vi "shag_start — 7.vi"() -> ()   [LabVIEW 2016]
uses:
  <vilib>/Instr/_visa.llb/VISA Configure Serial Port (Instr).vi
panel:
  out "file 2":string
  out "положение в мин 2":i32
  out "file":i32
  out "положение в мин 1":i32
  in  "all":T1(tab)
  out "положение шд 2":i32(knob) scale=-10.0..190.0
  out "текущее положение 2":string
  out "положение в минутах 2":string
  in  "Минуты 2":i32 min=-600 max=11400
  in  "Stop двигатель 2":bool
  in  "Вращение по градусам +  2":bool
  in  "Вращение по градусам -  2":bool
  in  "Вернуться в нулевое положение 2":bool
  in  "Задать текущее положение нулевым 2":bool
  in  "Установка минут 2":bool
  in  "Блокировать трубку №2":bool
  out "положение шд":i32(knob) scale=-10.0..190.0
  out "текущее положение":string
  out "положение в минутах 1":string
  in  "Минуты":i32 min=-600 max=11400
  in  "Stop двигатель":bool
  in  "Вращение по градусам +":bool
  in  "Вращение по градусам -":bool
  in  "Вернуться в нулевое положение":bool
  in  "Задать текущее положение нулевым":bool
  in  "Установка минут":bool
  in  "Блокировать зеркало №1":bool
  in  "stop":bool
  in  "Выберете COM порт":refnum<visa-resource-name>="COM1"
  in  "Скорость обмена данными":u32(ring)=19200 items=["9600"=9600, "19200"=19200, "38400"=38400, "57600"=57600]
  in  "Число бит на символ":u16=8 min=5 max=8 step=1
  in  "Контроль чётности":enum16{"None", "Odd", "Even", "Mark", "Space"}(ring)
  in  "Стоповый бит":u16(ring)=10 items=["1.0"=10, "1.5"=15, "2.0"=20]
  in  "Контроль переполнения":u16(ring) items=["None"=0, "XON/XOFF"=1, "RTS/CTS"=2, "DTR/DSR"=4]
  # "1 - адресс 1 двигателя\n2 - адресс 2 двигателя\n$0MV\\01+   - запуск всех двигателей в положительном направлении \n$0MS\\00   - остановка всех двигателей\n$0MJ\\04+\\00\\00\\01   - 1 шаг всех двигателей\n$0SS\\01\\10   - скорость 10 для всех двигателей"
  # "Ренгеновская трубка №2"
  # "Положение:"
  # "Зеркало №1"
  # "Положение:"
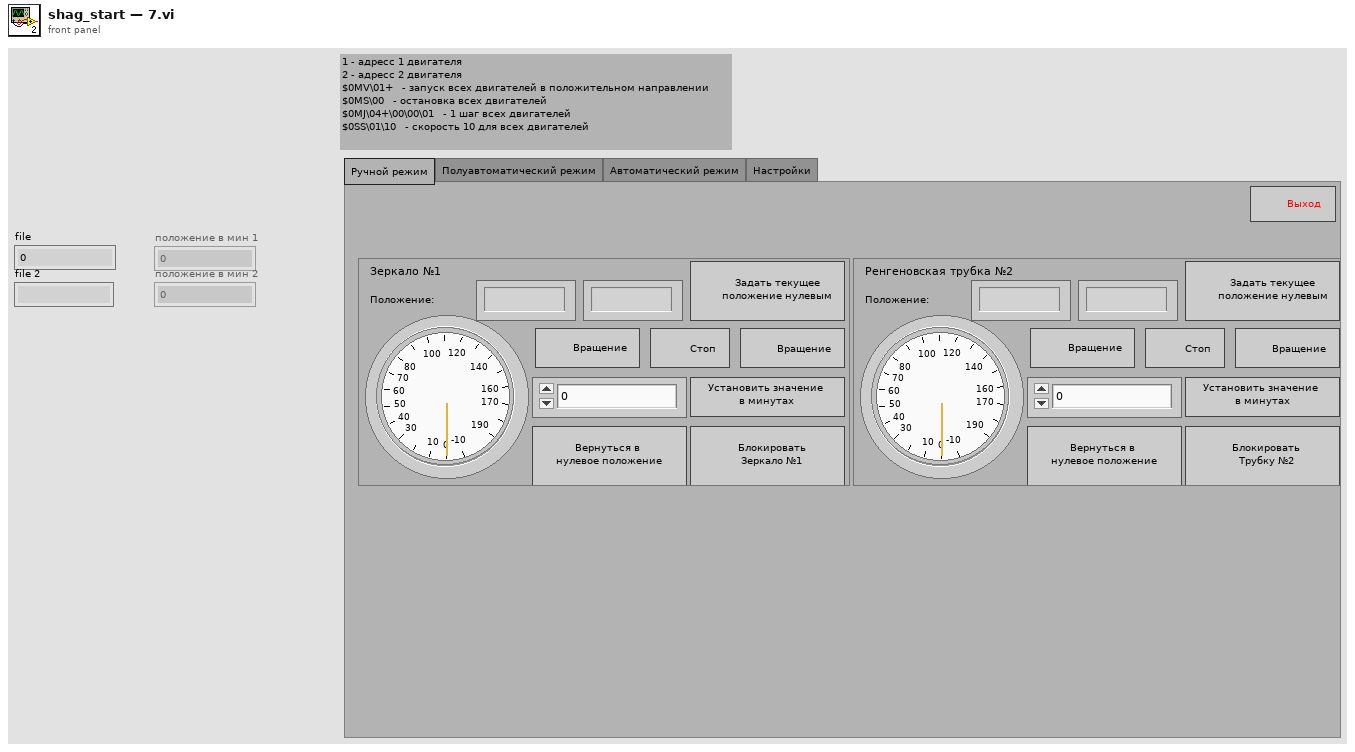
[diagram p1: front panel]
types:
  T1 = enum32{"Ручной режим", "Полуавтоматический режим", "Автоматический режим", "Настройки"}
  T2 = enum16{"open", "replace", "create", "open or create", "replace or create", "replace or create with confirmation"}
  T3 = enum8{"Enabled", "Disabled", "Disabled and Grayed Out"}
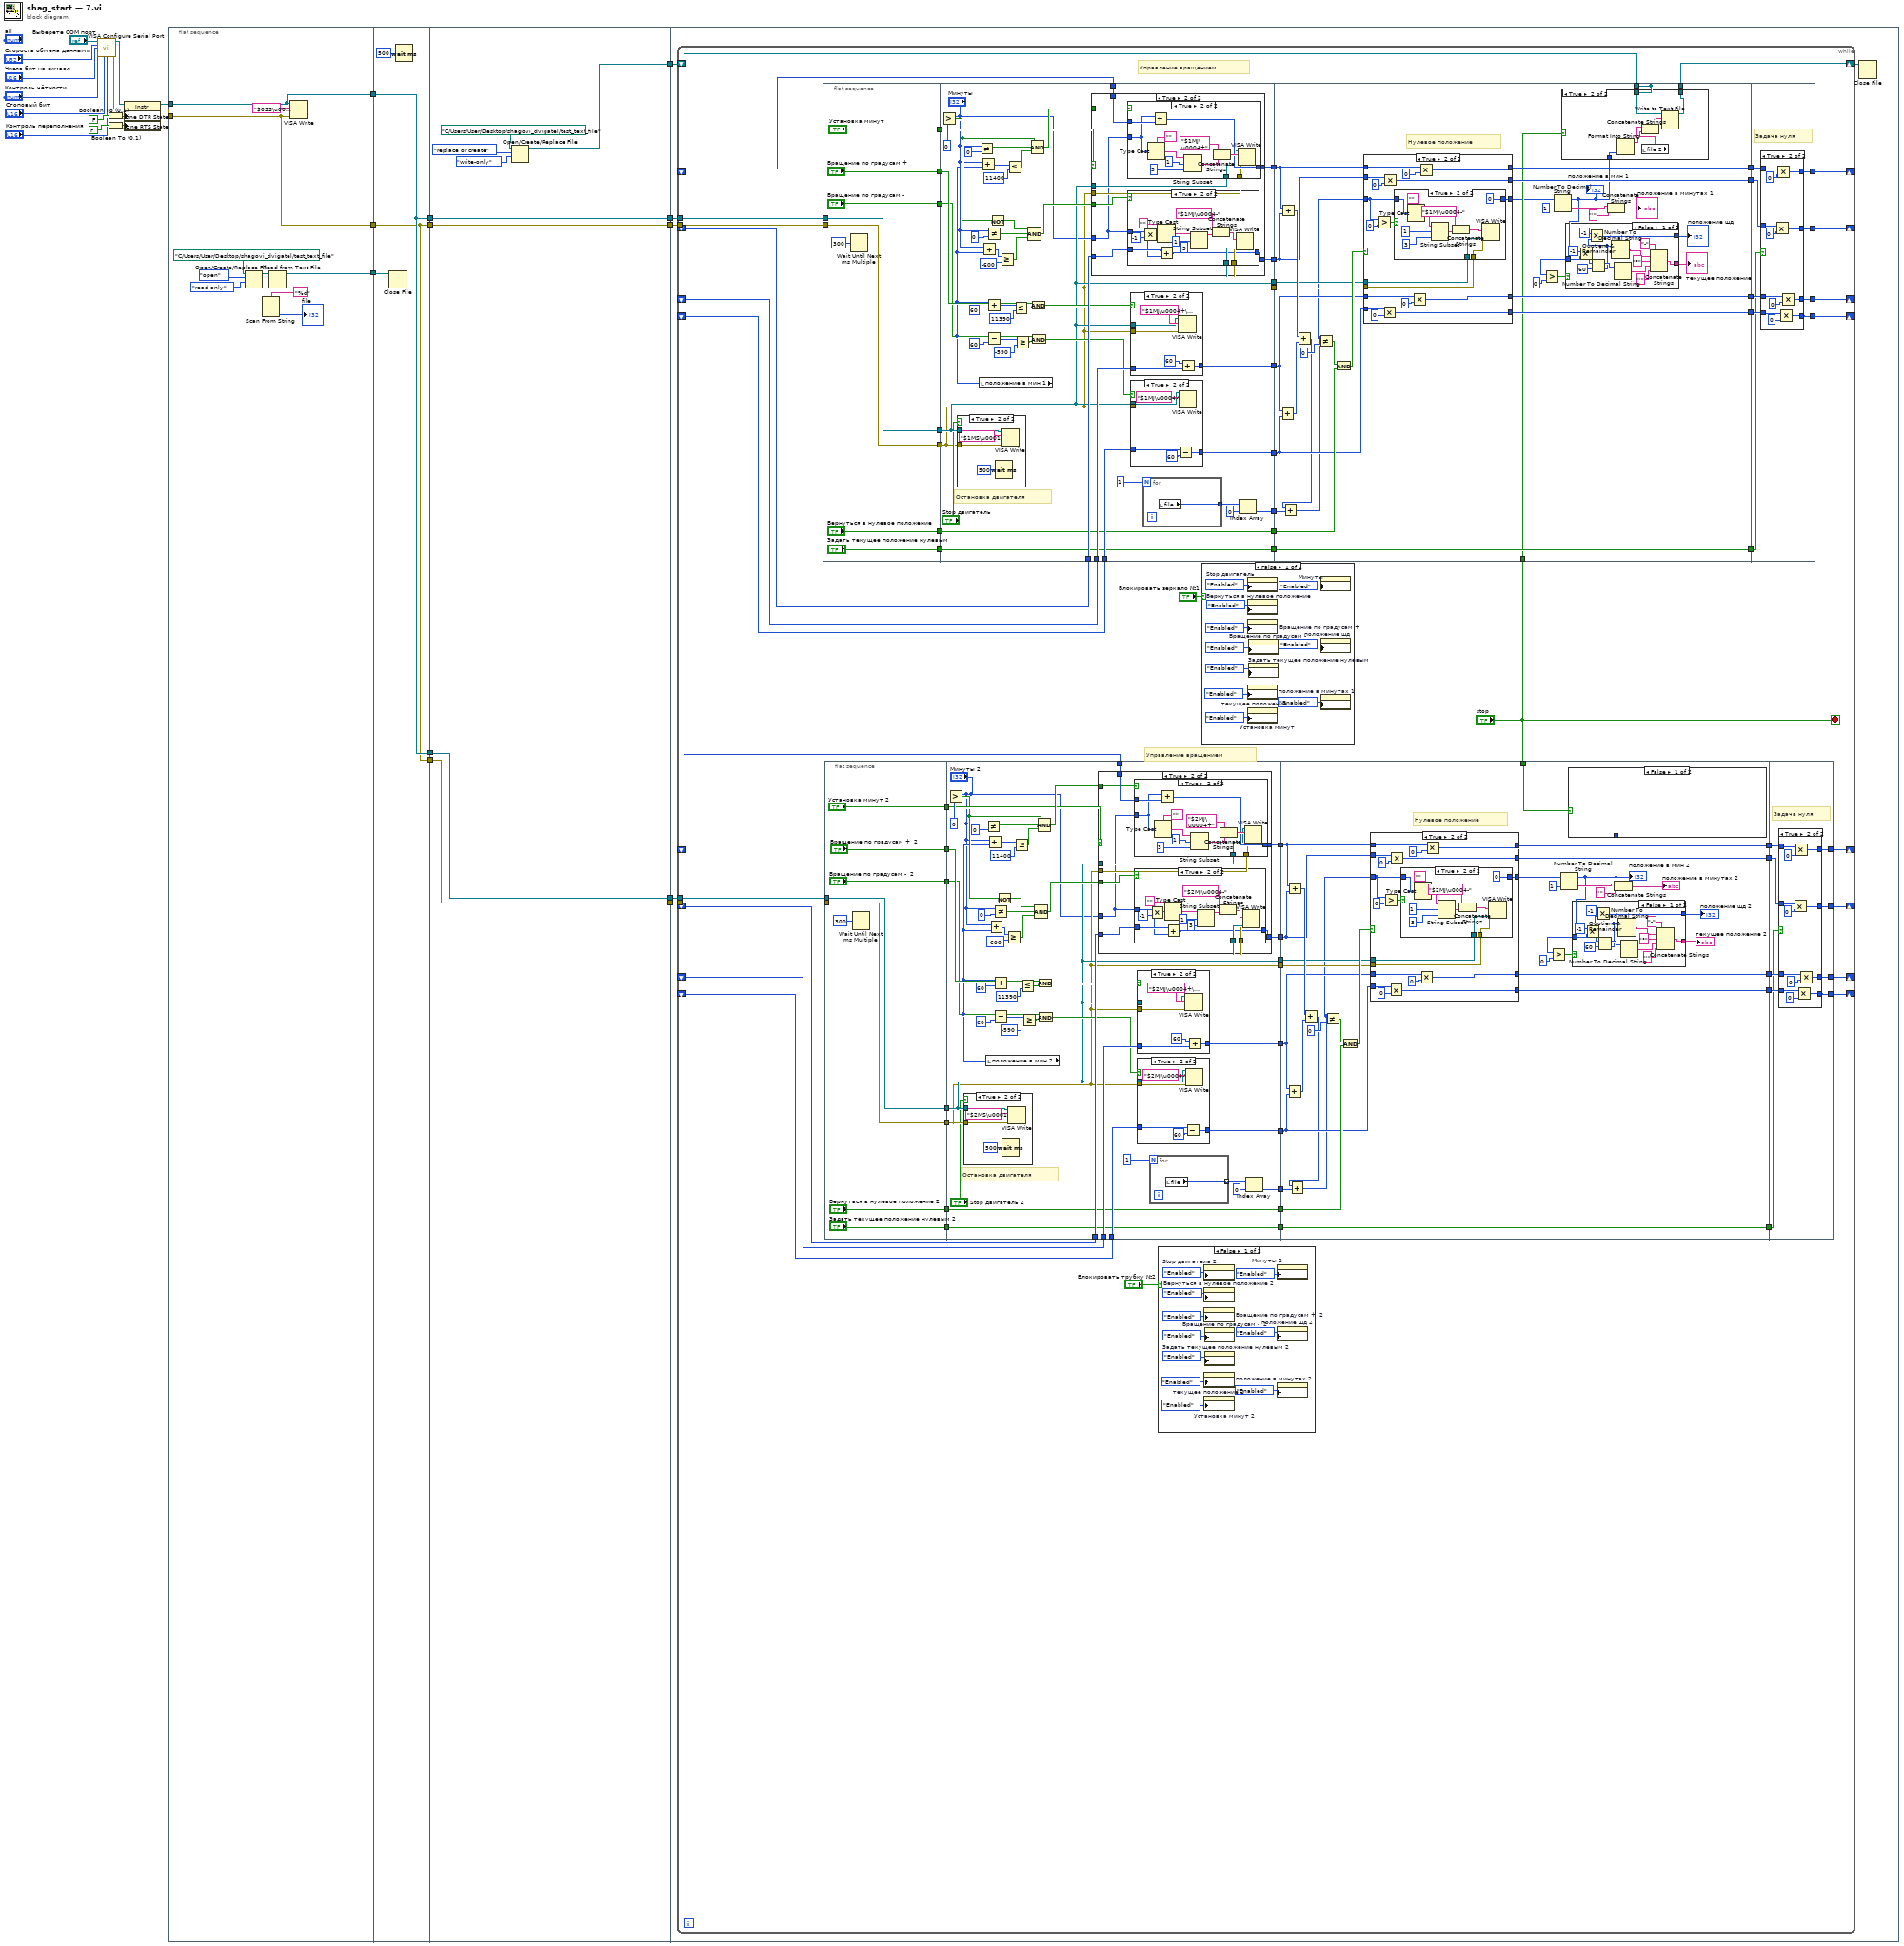
[diagram p0: block diagram]
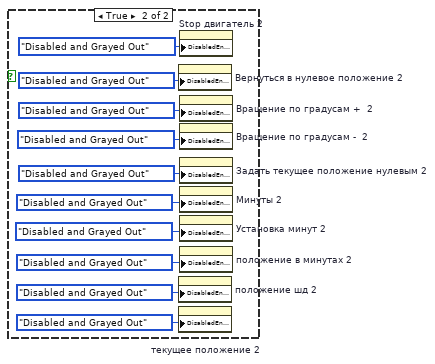
[diagram p2: hidden frame]
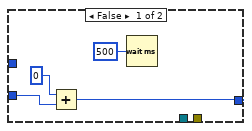
[diagram p4: hidden frame]
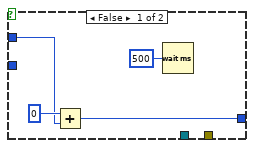
[diagram p5: hidden frame]
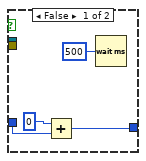
[diagram p7: hidden frame]
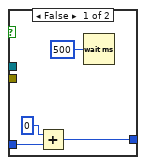
[diagram p8: hidden frame]
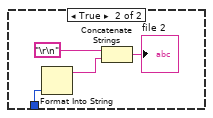
[diagram p9: hidden frame]
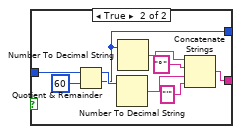
[diagram p10: hidden frame]
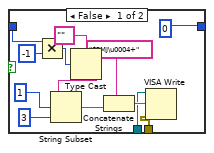
[diagram p12: hidden frame]
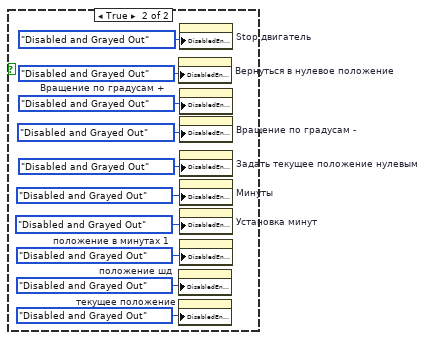
[diagram p14: hidden frame]
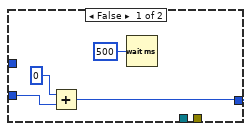
[diagram p16: hidden frame]
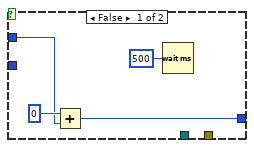
[diagram p17: hidden frame]
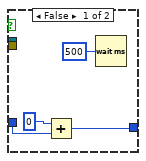
[diagram p19: hidden frame]
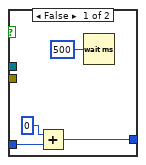
[diagram p20: hidden frame]
diagram:
  n1 = call-poly "VISA Configure Serial Port"("VISA resource name"="Выберете COM порт", "baud rate (9600)"="Скорость обмена данными", "data bits (8)"="Число бит на символ", "parity (0:none)"="Контроль чётности", "stop bits (10: 1 bit)"="Стоповый бит", "flow control (0:none)"="Контроль переполнения") -> ("VISA resource name out"=w24:refnum<visa-resource-name>, "error out"=w23:errorcluster)  [unwired: 8 in]
  n2 = Boolean To (0,1)(Boolean=FALSE ("DTR Write")) -> (0, 1=w25:i16)
  n3 = Boolean To (0,1)(Boolean=FALSE ("DTR Write")) -> (0, 1=w26:i16)
  n4 = property class="Instr"(reference=w24, error in=w23, "Serial Settings:Modem Line Settings:Line DTR State"=w25, "Serial Settings:Modem Line Settings:Line RTS State"=w26) -> (reference out=w22:refnum<visa-resource-name>, error out=w21:errorcluster)
  n5 = flat-sequence {
    tunnel: w22 -> [w36]
    tunnel: w21 -> [w35]
    tunnel: [w36] -> w20
    tunnel: [w35] -> w19
    tunnel: [w29] -> w10
    tunnel: [w40] -> w9
    tunnel: w20 -> [w40]
    tunnel: w19 -> [w39]
    tunnel: [w39] -> w7
    tunnel: [w40] -> w5
    tunnel: [w39] -> w3
    tunnel: w10 -> [w38]
    tunnel: w9 -> [w49]
    tunnel: [w49] -> w8
    tunnel: w7 -> [w48]
    tunnel: [w48] -> w6
    tunnel: w5 -> [w47]
    tunnel: [w47] -> w4
    tunnel: w3 -> [w46]
    tunnel: [w46] -> w2
    tunnel: [w42] -> w1
    tunnel: w8 -> [w55]
    tunnel: w6 -> [w54]
    tunnel: w4 -> [w50]
    tunnel: w2 -> [w53]
    tunnel: w1 -> [w52]
    frame #0 {
      n6 = Open/Create/Replace File(file path (use dialog)=path "C:/Users/User/Desktop/shagovi_dvigatel/test_text_file", operation (0:open)=T2."open", access (0:read/write)=enum16{"read/write", "read-only", "write-only"}."read-only") -> (refnum out=w28:refnum<file>)  [unwired: 3 in, 2 out]
      n7 = Read from Text File(file (use dialog)=w28) -> (refnum out=w29:refnum<file>, text=w32:string)  [unwired: 3 in, 2 out]
      n8 = Scan From String(format string="%d", input string=w32) -> (output 1=→"file":i32)  [unwired: 3 in, 3 out]
      n9 = VISA Write(VISA resource name=w36, write buffer="$0SS\u0001\u0010", error in (no error)=w35) -> ()  [unwired: 3 out]
    }
    frame #1 {
      n10 = Close File(refnum=w38) -> ()  [unwired: 1 in, 2 out]
      n11 = Wait (ms)(milliseconds to wait=u32 500) -> ()  [unwired: 1 out]
    }
    frame #2 {
      n12 = Open/Create/Replace File(file path (use dialog)=path "C:/Users/User/Desktop/shagovi_dvigatel/test_text_file", operation (0:open)=T2."replace or create", access (0:read/write)=enum16{"read/write", "read-only", "write-only"}."write-only") -> (refnum out=w42:refnum<file>)  [unwired: 3 in, 2 out]
    }
    frame #3 {
      n13 = while {
        tunnel: w55 -> [w98]
        tunnel: w54 -> [w97]
        shift-right: [w93] -> _
        shift-left: _ -> [w102]
        shift-right: [w94] -> _
        shift-left: _ -> [w101]
        shift-right: [w95] -> _
        shift-left: _ -> [w100]
        shift-right: [w96] -> _
        shift-left: _ -> [w99]
        tunnel: w53 -> [w67]
        shift-right: [w89] -> w51
        shift-left: w52 -> [w90]
        tunnel: w50 -> [w66]
        shift-right: [w62] -> _
        shift-left: _ -> [w63]
        shift-right: [w60] -> _
        shift-left: _ -> [w61]
        shift-right: [w58] -> _
        shift-left: _ -> [w59]
        shift-right: [w56] -> _
        shift-left: _ -> [w57]
        stop <- "stop" stop-if-true
        # "Управление вращением"
        # "Управление вращением"
        n14 = flat-sequence {
          tunnel: w97 -> [w423]
          tunnel: w98 -> [w424]
          tunnel: [w424] -> w122
          tunnel: [w423] -> w121
          tunnel: ["Вращение по градусам +"] -> w120
          tunnel: ["Вращение по градусам -"] -> w119
          tunnel: ["Вернуться в нулевое положение"] -> w118
          tunnel: ["Задать текущее положение нулевым"] -> w117
          tunnel: ["Установка минут"] -> w116
          tunnel: w122 -> [w448]
          tunnel: w121 -> [w430]
          tunnel: [w471] -> w115
          tunnel: w102 -> [w468]
          tunnel: w101 -> [w470]
          tunnel: [w469] -> w114
          tunnel: w100 -> [w467]
          tunnel: w99 -> [w466]
          tunnel: w120 -> [w452]
          tunnel: w119 -> [w451]
          tunnel: [w465] -> w113
          tunnel: [w464] -> w112
          tunnel: [w449] -> w111
          tunnel: w118 -> [w449]
          tunnel: [w430] -> w110
          tunnel: [w448] -> w109
          tunnel: [w447] -> w108
          tunnel: w117 -> [w447]
          tunnel: w116 -> [w441]
          tunnel: [w428] -> w91
          tunnel: w115 -> [w553]
          tunnel: w114 -> [w554]
          tunnel: [w573] -> w107
          tunnel: [w571] -> w106
          tunnel: w113 -> [w555]
          tunnel: w112 -> [w556]
          tunnel: [w562] -> w105
          tunnel: [w569] -> w104
          tunnel: w111 -> [w565]
          tunnel: w110 -> [w561]
          tunnel: w109 -> [w560]
          tunnel: w108 -> [w558]
          tunnel: [w558] -> w103
          tunnel: [w547] -> _
          tunnel: "stop" -> [w550]
          tunnel: w90 -> [w547]
          tunnel: w91 -> [w545]
          tunnel: [w542] -> w89
          tunnel: [w659] -> w93
          tunnel: [w656] -> w94
          tunnel: w107 -> [w658]
          tunnel: w106 -> [w657]
          tunnel: [w655] -> w95
          tunnel: [w654] -> w96
          tunnel: w105 -> [w653]
          tunnel: w104 -> [w652]
          tunnel: w103 -> [w651]
          frame #0 {
            n15 = Wait Until Next ms Multiple(millisecond multiple=u32 300) -> ()  [unwired: 1 out]
          }
          frame #1 {
            # "Остановка двигателя"
            n16 = Greater?(x="Минуты", y=0) -> (0:w439:bool)
            n17 = case shown="True" "Stop двигатель" {
              tunnel: w448 -> [_ w519]
              tunnel: w430 -> [_ w518]
              frame False {
              }
              frame True {
                n18 = Wait (ms)(milliseconds to wait=u32 500) -> ()  [unwired: 1 out]
                n19 = VISA Write(VISA resource name=w519, write buffer="$1MS\u0001", error in (no error)=w518) -> ()  [unwired: 3 out]
              }
            }
            n20 = Not Equal?(x="Минуты", y=0) -> (x != y?=w438:bool)
            n21 = local read "положение в мин 1"() -> (w429:i32)
            n22 = Add(x="Минуты", y=w429) -> (x+y=w462:i32)
            n23 = Add(x="Минуты", y=w429) -> (x+y=w433:i32)
            n24 = Not Equal?(x="Минуты", y=0) -> (x != y?=w436:bool)
            n25 = Add(x=w429, y=60) -> (x+y=w457:i32)
            n26 = Subtract(x=w429, y=60) -> (x-y=w444:i32)
            n27 = Not(x=w439) -> (.not. x?=w440:bool)
            n28 = Greater Or Equal?(x=w433, y=-600) -> (x >= y?=w434:bool)
            n29 = Less Or Equal?(x=w462, y=11400) -> (x <= y?=w437:bool)
            n30 = Less Or Equal?(x=w457, y=11390) -> (x <= y?=w454:bool)
            n31 = Greater Or Equal?(x=w444, y=-590) -> (x >= y?=w445:bool)
            n32 = Compound Arithmetic op=AND(w440, w436, w434) -> (w458:bool)
            n33 = And(x=w452, y=w454) -> (x .and. y?=w453:bool)
            n34 = And(x=w451, y=w445) -> (x .and. y?=w450:bool)
            n35 = Compound Arithmetic op=AND(w439, w438, w437) -> (w460:bool)
            n36 = case shown="True" w441 {
              tunnel: [w474 w483] -> w471
              tunnel: w470 -> [w473 w482]
              tunnel: [w473 w481] -> w469
              tunnel: w468 -> [w474 w480]
              tunnel: w460 -> [_ w479]
              tunnel: w458 -> [_ w478]
              tunnel: w430 -> [_ w477]
              tunnel: w448 -> [_ w476]
              tunnel: "Минуты" -> [_ w475]
              frame False {
              }
              frame True {
                n37 = case shown="True" w479 {
                  tunnel: [w504 w510] -> w483
                  tunnel: w480 -> [w503 w509]
                  tunnel: w477 -> [_ w508]
                  tunnel: w476 -> [_ w507]
                  tunnel: w475 -> [_ w506]
                  frame False {
                    n38 = Add(x=0, y=w503) -> (x+y=w504:i32)
                    n39 = Wait (ms)(milliseconds to wait=u32 500) -> ()  [unwired: 1 out]
                  }
                  frame True {
                    n40 = Type Cast(type="", x=w506) -> (*(type *) &x=w513:string)
                    n41 = Add(x=w506, y=w509) -> (x+y=w510:i32)
                    n42 = String Subset(string=w513, offset (0)=1, length (rest)=3 ("length (rest)")) -> (substring=w512:string)
                    n43 = Concatenate Strings("$1MJ\u0004+" ("write buffer"), w512) -> (w516:string)
                    n44 = VISA Write(VISA resource name=w507, write buffer=w516, error in (no error)=w508) -> ()  [unwired: 3 out]
                  }
                }
                n45 = case shown="True" w478 {
                  tunnel: [w486 w492] -> w481
                  tunnel: w482 -> [w485 w491]
                  tunnel: w476 -> [_ w494]
                  tunnel: w477 -> [_ w493]
                  tunnel: w475 -> [_ w488]
                  frame False {
                    n46 = Add(x=0, y=w485) -> (x+y=w486:i32)
                    n47 = Wait (ms)(milliseconds to wait=u32 500) -> ()  [unwired: 1 out]
                  }
                  frame True {
                    n48 = Multiply(x=w488, y=-1) -> (x*y=w490:i32)
                    n49 = Type Cast(type="", x=w490) -> (*(type *) &x=w497:string)
                    n50 = Add(x=w491, y=w488) -> (x+y=w492:i32)
                    n51 = String Subset(string=w497, offset (0)=1, length (rest)=3 ("length (rest)")) -> (substring=w496:string)
                    n52 = Concatenate Strings("$1MJ\u0004-" ("write buffer"), w496) -> (w500:string)
                    n53 = VISA Write(VISA resource name=w494, write buffer=w500, error in (no error)=w493) -> ()  [unwired: 3 out]
                  }
                }
              }
            }
            n54 = case shown="True" w453 {
              tunnel: [w534 w541] -> w465
              tunnel: w467 -> [w533 w536]
              tunnel: w448 -> [_ w537]
              tunnel: w430 -> [_ w538]
              frame False {
                n55 = Add(x=0, y=w533) -> (x+y=w534:i32)
                n56 = Wait (ms)(milliseconds to wait=u32 500) -> ()  [unwired: 1 out]
              }
              frame True {
                n57 = VISA Write(VISA resource name=w537, write buffer="$1MJ\u0004+\u0000\u0000<", error in (no error)=w538) -> ()  [unwired: 3 out]
                n58 = Add(x=60, y=w536) -> (x+y=w541:i32)
              }
            }
            n59 = case shown="True" w450 {
              tunnel: [w524 w527] -> w464
              tunnel: w466 -> [w523 w526]
              tunnel: w448 -> [_ w530]
              tunnel: w430 -> [_ w529]
              frame False {
                n60 = Add(x=0, y=w523) -> (x+y=w524:i32)
                n61 = Wait (ms)(milliseconds to wait=u32 500) -> ()  [unwired: 1 out]
              }
              frame True {
                n62 = Subtract(x=w526, y=60 ("x")) -> (x-y=w527:i32)
                n63 = VISA Write(VISA resource name=w530, write buffer="$1MJ\u0004-\u0000\u0000<", error in (no error)=w529) -> ()  [unwired: 3 out]
              }
            }
            n64 = for {
              N: 1 -> [_]
              tunnel: [w472] -> w426 mode=indexing
              n65 = local read "file"() -> (w472:i32)
            }
            n66 = Index Array(array=w426, index=0) -> (element=w428:i32)
          }
          frame #2 {
            # "Нулевое положение"
            n67 = Add(x=w555, y=w556) -> (x+y=w566:i32)
            n68 = Add(x=w553, y=w554) -> (x+y=w570:i32)
            n69 = Add(x=w570, y=w566) -> (x+y=w544:i32)
            n70 = Add(x=w544, y=w545) -> (x+y=w543:i32)
            n71 = Not Equal?(x=w543, y=0 ("x")) -> (x != y?=w563:bool)
            n72 = And(x=w563, y=w565) -> (x .and. y?=w572:bool)
            n73 = case shown="True" w572 {
              tunnel: [w604 w626] -> w546
              tunnel: w553 -> [w608 w623]
              tunnel: [w608 w622] -> w573
              tunnel: [w607 w621] -> w571
              tunnel: w543 -> [w604 w615]
              tunnel: [w605 w617] -> w569
              tunnel: [w606 w614] -> w562
              tunnel: w554 -> [w607 w613]
              tunnel: w561 -> [_ w612]
              tunnel: w560 -> [_ w611]
              tunnel: w555 -> [w606 w610]
              tunnel: w556 -> [w605 w609]
              frame False {
              }
              frame True {
                n74 = Greater?(x=w615, y=0) -> (0:w616:bool)
                n75 = Multiply(x=w609, y=0) -> (x*y=w617:i32)
                n76 = Multiply(x=w613, y=0) -> (x*y=w621:i32)
                n77 = case shown="True" w616 {
                  tunnel: w615 -> [w631 w644]
                  tunnel: [0 0] -> w626
                  tunnel: w611 -> [w628 w641]
                  tunnel: w612 -> [w627 w640]
                  frame False {
                    n78 = Multiply(x=w631, y=-1) -> (x*y=w629:i32)
                    n79 = Type Cast(type="", x=w629) -> (*(type *) &x=w635:string)
                    n80 = String Subset(string=w635, offset (0)=1, length (rest)=3 ("length (rest)")) -> (substring=w634:string)
                    n81 = Concatenate Strings("$1MJ\u0004+" ("write buffer"), w634) -> (w638:string)
                    n82 = VISA Write(VISA resource name=w628, write buffer=w638, error in (no error)=w627) -> ()  [unwired: 3 out]
                  }
                  frame True {
                    n83 = Type Cast(type="", x=w644) -> (*(type *) &x=w647:string)
                    n84 = String Subset(string=w647, offset (0)=1, length (rest)=3 ("length (rest)")) -> (substring=w646:string)
                    n85 = Concatenate Strings("$1MJ\u0004-" ("write buffer"), w646) -> (w642:string)
                    n86 = VISA Write(VISA resource name=w641, write buffer=w642, error in (no error)=w640) -> ()  [unwired: 3 out]
                  }
                }
                n87 = Multiply(x=w610, y=0) -> (x*y=w614:i32)
                n88 = Multiply(x=w623, y=0) -> (x*y=w622:i32)
              }
            }
            "положение в мин 1" <- w546
            n89 = Greater?(x=w546, y=0) -> (0:w568:bool)
            n90 = Number To Decimal String(number=w546, width (-)=i16 1) -> (decimal integer string=w549:string)
            n91 = case shown="True" w550 {
              tunnel: w547 -> [w574 w579]
              tunnel: w546 -> [_ w580]
              tunnel: [w574 w578] -> w542
              frame False {
              }
              frame True {
                n92 = Format Into String(w580) -> (resulting string=w576:string)  [unwired: 3 in, 1 out]
                n93 = local read "file 2"() -> (w575:string)
                n94 = Concatenate Strings(w576, w575) -> (w577:string)
                n95 = Write to Text File(file (use dialog)=w579, text=w577) -> (refnum out=w578:refnum<file>)  [unwired: 2 in, 2 out]
              }
            }
            n96 = case shown="False" w568 {
              tunnel: w546 -> [w587 w603]
              tunnel: [w591 w597] -> w559
              tunnel: [w581 w595] -> w557
              frame False {
                n97 = Multiply(x=-1, y=w587) -> (x*y=w586:i32)
                n98 = Quotient & Remainder(x=w586, y=60) -> (x-y*floor(x/y)=w590:i32, floor(x/y)=w582:i32)
                n99 = Multiply(x=-1, y=w582) -> (x*y=w581:i32)
                n100 = Number To Decimal String(number=w582) -> (decimal integer string=w588:string)  [unwired: 1 in]
                n101 = Number To Decimal String(number=w590) -> (decimal integer string=w589:string)  [unwired: 1 in]
                n102 = Concatenate Strings("-" ("string"), w588, "°" ("string"), w589, "'" ("string")) -> (w591:string)
              }
              frame True {
                n103 = Quotient & Remainder(x=w603, y=60) -> (x-y*floor(x/y)=w596:i32, floor(x/y)=w595:i32)
                n104 = Number To Decimal String(number=w596) -> (decimal integer string=w598:string)  [unwired: 1 in]
                n105 = Number To Decimal String(number=w595) -> (decimal integer string=w599:string)  [unwired: 1 in]
                n106 = Concatenate Strings(w599, "°" ("string"), w598, "'" ("string")) -> (w597:string)
              }
            }
            "положение шд" <- w557
            "текущее положение" <- w559
            n107 = Concatenate Strings(w549, "'" ("string")) -> (→"положение в минутах 1":string)
          }
          frame #3 {
            # "Задача нуля"
            n108 = case shown="True" w651 {
              tunnel: [w663 w674] -> w659
              tunnel: w658 -> [w663 w675]
              tunnel: w657 -> [w662 w671]
              tunnel: [w662 w670] -> w656
              tunnel: [w661 w667] -> w655
              tunnel: [w660 w666] -> w654
              tunnel: w653 -> [w661 w665]
              tunnel: w652 -> [w660 w664]
              frame False {
              }
              frame True {
                n109 = Multiply(x=w671, y=0) -> (x*y=w670:i32)
                n110 = Multiply(x=w675, y=0) -> (x*y=w674:i32)
                n111 = Multiply(x=w664, y=0) -> (x*y=w666:i32)
                n112 = Multiply(x=w665, y=0) -> (x*y=w667:i32)
              }
            }
          }
        }
        n113 = flat-sequence {
          tunnel: w67 -> [w149]
          tunnel: w66 -> [w150]
          tunnel: [w150] -> w88
          tunnel: [w149] -> w87
          tunnel: ["Вращение по градусам +  2"] -> w86
          tunnel: ["Вращение по градусам -  2"] -> w85
          tunnel: ["Вернуться в нулевое положение 2"] -> w84
          tunnel: ["Задать текущее положение нулевым 2"] -> w83
          tunnel: ["Установка минут 2"] -> w82
          tunnel: w88 -> [w174]
          tunnel: w87 -> [w158]
          tunnel: [w197] -> w81
          tunnel: w63 -> [w194]
          tunnel: w61 -> [w196]
          tunnel: [w195] -> w80
          tunnel: w59 -> [w193]
          tunnel: w57 -> [w192]
          tunnel: w86 -> [w178]
          tunnel: w85 -> [w177]
          tunnel: [w191] -> w79
          tunnel: [w190] -> w78
          tunnel: [w175] -> w77
          tunnel: w84 -> [w175]
          tunnel: [w158] -> w76
          tunnel: [w174] -> w75
          tunnel: [w173] -> w74
          tunnel: w83 -> [w173]
          tunnel: w82 -> [w167]
          tunnel: [w156] -> w73
          tunnel: w81 -> [w279]
          tunnel: w80 -> [w280]
          tunnel: [w297] -> w72
          tunnel: [w295] -> w71
          tunnel: w79 -> [w281]
          tunnel: w78 -> [w282]
          tunnel: [w286] -> w70
          tunnel: [w293] -> w69
          tunnel: w77 -> [w289]
          tunnel: w76 -> [w285]
          tunnel: w75 -> [w284]
          tunnel: w74 -> [w283]
          tunnel: [w283] -> w68
          tunnel: w73 -> [w275]
          tunnel: "stop" -> [w270]
          tunnel: [w380] -> w62
          tunnel: [w377] -> w60
          tunnel: w72 -> [w379]
          tunnel: w71 -> [w378]
          tunnel: [w376] -> w58
          tunnel: [w375] -> w56
          tunnel: w70 -> [w374]
          tunnel: w69 -> [w373]
          tunnel: w68 -> [w372]
          frame #0 {
            n114 = Wait Until Next ms Multiple(millisecond multiple=u32 300) -> ()  [unwired: 1 out]
          }
          frame #1 {
            # "Остановка двигателя"
            n115 = Greater?(x="Минуты 2", y=0) -> (0:w165:bool)
            n116 = case shown="True" "Stop двигатель 2" {
              tunnel: w174 -> [_ w245]
              tunnel: w158 -> [_ w244]
              frame False {
              }
              frame True {
                n117 = Wait (ms)(milliseconds to wait=u32 500) -> ()  [unwired: 1 out]
                n118 = VISA Write(VISA resource name=w245, write buffer="$2MS\u0001", error in (no error)=w244) -> ()  [unwired: 3 out]
              }
            }
            n119 = Not Equal?(x="Минуты 2", y=0) -> (x != y?=w164:bool)
            n120 = local read "положение в мин 2"() -> (w157:i32)
            n121 = Add(x="Минуты 2", y=w157) -> (x+y=w188:i32)
            n122 = Add(x="Минуты 2", y=w157) -> (x+y=w160:i32)
            n123 = Not Equal?(x="Минуты 2", y=0) -> (x != y?=w162:bool)
            n124 = Add(x=w157, y=60) -> (x+y=w183:i32)
            n125 = Subtract(x=w157, y=60) -> (x-y=w170:i32)
            n126 = Not(x=w165) -> (.not. x?=w166:bool)
            n127 = Greater Or Equal?(x=w160, y=-600) -> (x >= y?=w161:bool)
            n128 = Less Or Equal?(x=w188, y=11400) -> (x <= y?=w163:bool)
            n129 = Less Or Equal?(x=w183, y=11390) -> (x <= y?=w180:bool)
            n130 = Greater Or Equal?(x=w170, y=-590) -> (x >= y?=w171:bool)
            n131 = Compound Arithmetic op=AND(w166, w162, w161) -> (w184:bool)
            n132 = And(x=w178, y=w180) -> (x .and. y?=w179:bool)
            n133 = And(x=w177, y=w171) -> (x .and. y?=w176:bool)
            n134 = Compound Arithmetic op=AND(w165, w164, w163) -> (w186:bool)
            n135 = case shown="True" w167 {
              tunnel: [w200 w209] -> w197
              tunnel: w196 -> [w199 w208]
              tunnel: [w199 w207] -> w195
              tunnel: w194 -> [w200 w206]
              tunnel: w186 -> [_ w205]
              tunnel: w184 -> [_ w204]
              tunnel: w158 -> [_ w203]
              tunnel: w174 -> [_ w202]
              tunnel: "Минуты 2" -> [_ w201]
              frame False {
              }
              frame True {
                n136 = case shown="True" w205 {
                  tunnel: [w230 w236] -> w209
                  tunnel: w206 -> [w229 w235]
                  tunnel: w203 -> [_ w234]
                  tunnel: w202 -> [_ w233]
                  tunnel: w201 -> [_ w232]
                  frame False {
                    n137 = Add(x=0, y=w229) -> (x+y=w230:i32)
                    n138 = Wait (ms)(milliseconds to wait=u32 500) -> ()  [unwired: 1 out]
                  }
                  frame True {
                    n139 = Type Cast(type="", x=w232) -> (*(type *) &x=w239:string)
                    n140 = Add(x=w232, y=w235) -> (x+y=w236:i32)
                    n141 = String Subset(string=w239, offset (0)=1, length (rest)=3 ("length (rest)")) -> (substring=w238:string)
                    n142 = Concatenate Strings("$2MJ\u0004+" ("write buffer"), w238) -> (w242:string)
                    n143 = VISA Write(VISA resource name=w233, write buffer=w242, error in (no error)=w234) -> ()  [unwired: 3 out]
                  }
                }
                n144 = case shown="True" w204 {
                  tunnel: [w212 w218] -> w207
                  tunnel: w208 -> [w211 w217]
                  tunnel: w202 -> [_ w220]
                  tunnel: w203 -> [_ w219]
                  tunnel: w201 -> [_ w214]
                  frame False {
                    n145 = Add(x=0, y=w211) -> (x+y=w212:i32)
                    n146 = Wait (ms)(milliseconds to wait=u32 500) -> ()  [unwired: 1 out]
                  }
                  frame True {
                    n147 = Multiply(x=w214, y=-1) -> (x*y=w216:i32)
                    n148 = Type Cast(type="", x=w216) -> (*(type *) &x=w223:string)
                    n149 = Add(x=w217, y=w214) -> (x+y=w218:i32)
                    n150 = String Subset(string=w223, offset (0)=1, length (rest)=3 ("length (rest)")) -> (substring=w222:string)
                    n151 = Concatenate Strings("$2MJ\u0004-" ("write buffer"), w222) -> (w226:string)
                    n152 = VISA Write(VISA resource name=w220, write buffer=w226, error in (no error)=w219) -> ()  [unwired: 3 out]
                  }
                }
              }
            }
            n153 = case shown="True" w179 {
              tunnel: [w260 w267] -> w191
              tunnel: w193 -> [w259 w262]
              tunnel: w174 -> [_ w263]
              tunnel: w158 -> [_ w264]
              frame False {
                n154 = Add(x=0, y=w259) -> (x+y=w260:i32)
                n155 = Wait (ms)(milliseconds to wait=u32 500) -> ()  [unwired: 1 out]
              }
              frame True {
                n156 = VISA Write(VISA resource name=w263, write buffer="$2MJ\u0004+\u0000\u0000<", error in (no error)=w264) -> ()  [unwired: 3 out]
                n157 = Add(x=60, y=w262) -> (x+y=w267:i32)
              }
            }
            n158 = case shown="True" w176 {
              tunnel: [w250 w253] -> w190
              tunnel: w192 -> [w249 w252]
              tunnel: w174 -> [_ w256]
              tunnel: w158 -> [_ w255]
              frame False {
                n159 = Add(x=0, y=w249) -> (x+y=w250:i32)
                n160 = Wait (ms)(milliseconds to wait=u32 500) -> ()  [unwired: 1 out]
              }
              frame True {
                n161 = Subtract(x=w252, y=60 ("x")) -> (x-y=w253:i32)
                n162 = VISA Write(VISA resource name=w256, write buffer="$2MJ\u0004-\u0000\u0000<", error in (no error)=w255) -> ()  [unwired: 3 out]
              }
            }
            n163 = for {
              N: 1 -> [_]
              tunnel: [w198] -> w154 mode=indexing
              n164 = local read "file"() -> (w198:i32)
            }
            n165 = Index Array(array=w154, index=0) -> (element=w156:i32)
          }
          frame #2 {
            # "Нулевое положение"
            n166 = Add(x=w281, y=w282) -> (x+y=w290:i32)
            n167 = Add(x=w279, y=w280) -> (x+y=w294:i32)
            n168 = Add(x=w294, y=w290) -> (x+y=w274:i32)
            n169 = Add(x=w274, y=w275) -> (x+y=w273:i32)
            n170 = Not Equal?(x=w273, y=0 ("x")) -> (x != y?=w287:bool)
            n171 = And(x=w287, y=w289) -> (x .and. y?=w296:bool)
            n172 = case shown="True" w296 {
              tunnel: [w325 w347] -> w268
              tunnel: w279 -> [w329 w344]
              tunnel: [w329 w343] -> w297
              tunnel: [w328 w342] -> w295
              tunnel: w273 -> [w325 w336]
              tunnel: [w326 w338] -> w293
              tunnel: [w327 w335] -> w286
              tunnel: w280 -> [w328 w334]
              tunnel: w285 -> [_ w333]
              tunnel: w284 -> [_ w332]
              tunnel: w281 -> [w327 w331]
              tunnel: w282 -> [w326 w330]
              frame False {
              }
              frame True {
                n173 = Greater?(x=w336, y=0) -> (0:w337:bool)
                n174 = Multiply(x=w330, y=0) -> (x*y=w338:i32)
                n175 = Multiply(x=w334, y=0) -> (x*y=w342:i32)
                n176 = case shown="True" w337 {
                  tunnel: w336 -> [w352 w365]
                  tunnel: [0 0] -> w347
                  tunnel: w332 -> [w349 w362]
                  tunnel: w333 -> [w348 w361]
                  frame False {
                    n177 = Multiply(x=w352, y=-1) -> (x*y=w350:i32)
                    n178 = Type Cast(type="", x=w350) -> (*(type *) &x=w356:string)
                    n179 = String Subset(string=w356, offset (0)=1, length (rest)=3 ("length (rest)")) -> (substring=w355:string)
                    n180 = Concatenate Strings("$2MJ\u0004+" ("write buffer"), w355) -> (w359:string)
                    n181 = VISA Write(VISA resource name=w349, write buffer=w359, error in (no error)=w348) -> ()  [unwired: 3 out]
                  }
                  frame True {
                    n182 = Type Cast(type="", x=w365) -> (*(type *) &x=w368:string)
                    n183 = String Subset(string=w368, offset (0)=1, length (rest)=3 ("length (rest)")) -> (substring=w367:string)
                    n184 = Concatenate Strings("$2MJ\u0004-" ("write buffer"), w367) -> (w363:string)
                    n185 = VISA Write(VISA resource name=w362, write buffer=w363, error in (no error)=w361) -> ()  [unwired: 3 out]
                  }
                }
                n186 = Multiply(x=w331, y=0) -> (x*y=w335:i32)
                n187 = Multiply(x=w344, y=0) -> (x*y=w343:i32)
              }
            }
            "положение в мин 2" <- w268
            n188 = Greater?(x=w268, y=0) -> (0:w292:bool)
            n189 = Number To Decimal String(number=w268, width (-)=i16 1) -> (decimal integer string=w277:string)
            n190 = case shown="False" w270 {
              tunnel: w268 -> [_ w301]
              frame False {
              }
              frame True {
                n191 = Format Into String(w301) -> (resulting string=w299:string)  [unwired: 3 in, 1 out]
                n192 = Concatenate Strings("\r\n", w299) -> (→"file 2":string)
              }
            }
            n193 = case shown="False" w292 {
              tunnel: w268 -> [w308 w324]
              tunnel: [w312 w318] -> w271
              tunnel: [w302 w316] -> w269
              frame False {
                n194 = Multiply(x=-1, y=w308) -> (x*y=w307:i32)
                n195 = Quotient & Remainder(x=w307, y=60) -> (x-y*floor(x/y)=w311:i32, floor(x/y)=w303:i32)
                n196 = Multiply(x=-1, y=w303) -> (x*y=w302:i32)
                n197 = Number To Decimal String(number=w303) -> (decimal integer string=w309:string)  [unwired: 1 in]
                n198 = Number To Decimal String(number=w311) -> (decimal integer string=w310:string)  [unwired: 1 in]
                n199 = Concatenate Strings("-" ("string"), w309, "°" ("string"), w310, "'" ("string")) -> (w312:string)
              }
              frame True {
                n200 = Quotient & Remainder(x=w324, y=60) -> (x-y*floor(x/y)=w317:i32, floor(x/y)=w316:i32)
                n201 = Number To Decimal String(number=w317) -> (decimal integer string=w319:string)  [unwired: 1 in]
                n202 = Number To Decimal String(number=w316) -> (decimal integer string=w320:string)  [unwired: 1 in]
                n203 = Concatenate Strings(w320, "°" ("string"), w319, "'" ("string")) -> (w318:string)
              }
            }
            "положение шд 2" <- w269
            "текущее положение 2" <- w271
            n204 = Concatenate Strings(w277, "'" ("string")) -> (→"положение в минутах 2":string)
          }
          frame #3 {
            # "Задача нуля"
            n205 = case shown="True" w372 {
              tunnel: [w384 w395] -> w380
              tunnel: w379 -> [w384 w396]
              tunnel: w378 -> [w383 w392]
              tunnel: [w383 w391] -> w377
              tunnel: [w382 w388] -> w376
              tunnel: [w381 w387] -> w375
              tunnel: w374 -> [w382 w386]
              tunnel: w373 -> [w381 w385]
              frame False {
              }
              frame True {
                n206 = Multiply(x=w392, y=0) -> (x*y=w391:i32)
                n207 = Multiply(x=w396, y=0) -> (x*y=w395:i32)
                n208 = Multiply(x=w385, y=0) -> (x*y=w387:i32)
                n209 = Multiply(x=w386, y=0) -> (x*y=w388:i32)
              }
            }
          }
        }
        n210 = case shown="False" "Блокировать трубку №2" {
          frame False {
            n211 = property on="Stop двигатель 2" class="Bool"("DisabledEnum"=T3."Enabled" ("Disabled")) -> ()  [unwired: 2 in, 2 out]
            n212 = property on="Вернуться в нулевое положение 2" class="Bool"("DisabledEnum"=T3."Enabled" ("Disabled")) -> ()  [unwired: 2 in, 2 out]
            n213 = property on="Вращение по градусам +  2" class="Bool"("DisabledEnum"=T3."Enabled" ("Disabled")) -> ()  [unwired: 2 in, 2 out]
            n214 = property on="текущее положение 2" class="Str"("DisabledEnum"=T3."Enabled" ("Disabled")) -> ()  [unwired: 2 in, 2 out]
            n215 = property on="Установка минут 2" class="Bool"("DisabledEnum"=T3."Enabled" ("Disabled")) -> ()  [unwired: 2 in, 2 out]
            n216 = property on="Вращение по градусам -  2" class="Bool"("DisabledEnum"=T3."Enabled" ("Disabled")) -> ()  [unwired: 2 in, 2 out]
            n217 = property on="Задать текущее положение нулевым 2" class="Bool"("DisabledEnum"=T3."Enabled" ("Disabled")) -> ()  [unwired: 2 in, 2 out]
            n218 = property on="Минуты 2" class="DigNum (strict)"("DisabledEnum"=T3."Enabled" ("Disabled")) -> ()  [unwired: 2 in, 2 out]
            n219 = property on="положение шд 2" class="Knob (strict)"("DisabledEnum"=T3."Enabled" ("Disabled")) -> ()  [unwired: 2 in, 2 out]
            n220 = property on="положение в минутах 2" class="Str"("DisabledEnum"=T3."Enabled" ("Disabled")) -> ()  [unwired: 2 in, 2 out]
          }
          frame True {
            n221 = property on="Вернуться в нулевое положение 2" class="Bool"("DisabledEnum"=T3."Disabled and Grayed Out" ("Disabled")) -> ()  [unwired: 2 in, 2 out]
            n222 = property on="положение шд 2" class="Knob (strict)"("DisabledEnum"=T3."Disabled and Grayed Out" ("Disabled")) -> ()  [unwired: 2 in, 2 out]
            n223 = property on="текущее положение 2" class="Str"("DisabledEnum"=T3."Disabled and Grayed Out" ("Disabled")) -> ()  [unwired: 2 in, 2 out]
            n224 = property on="Stop двигатель 2" class="Bool"("DisabledEnum"=T3."Disabled and Grayed Out" ("Disabled")) -> ()  [unwired: 2 in, 2 out]
            n225 = property on="Вращение по градусам +  2" class="Bool"("DisabledEnum"=T3."Disabled and Grayed Out" ("Disabled")) -> ()  [unwired: 2 in, 2 out]
            n226 = property on="Вращение по градусам -  2" class="Bool"("DisabledEnum"=T3."Disabled and Grayed Out" ("Disabled")) -> ()  [unwired: 2 in, 2 out]
            n227 = property on="Задать текущее положение нулевым 2" class="Bool"("DisabledEnum"=T3."Disabled and Grayed Out" ("Disabled")) -> ()  [unwired: 2 in, 2 out]
            n228 = property on="Минуты 2" class="DigNum (strict)"("DisabledEnum"=T3."Disabled and Grayed Out" ("Disabled")) -> ()  [unwired: 2 in, 2 out]
            n229 = property on="Установка минут 2" class="Bool"("DisabledEnum"=T3."Disabled and Grayed Out" ("Disabled")) -> ()  [unwired: 2 in, 2 out]
            n230 = property on="положение в минутах 2" class="Str"("DisabledEnum"=T3."Disabled and Grayed Out" ("Disabled")) -> ()  [unwired: 2 in, 2 out]
          }
        }
        n231 = case shown="False" "Блокировать зеркало №1" {
          frame False {
            n232 = property on="Stop двигатель" class="Bool"("DisabledEnum"=T3."Enabled" ("Disabled")) -> ()  [unwired: 2 in, 2 out]
            n233 = property on="Вернуться в нулевое положение" class="Bool"("DisabledEnum"=T3."Enabled" ("Disabled")) -> ()  [unwired: 2 in, 2 out]
            n234 = property on="Вращение по градусам +" class="Bool"("DisabledEnum"=T3."Enabled" ("Disabled")) -> ()  [unwired: 2 in, 2 out]
            n235 = property on="текущее положение" class="Str"("DisabledEnum"=T3."Enabled" ("Disabled")) -> ()  [unwired: 2 in, 2 out]
            n236 = property on="Установка минут" class="Bool"("DisabledEnum"=T3."Enabled" ("Disabled")) -> ()  [unwired: 2 in, 2 out]
            n237 = property on="Вращение по градусам -" class="Bool"("DisabledEnum"=T3."Enabled" ("Disabled")) -> ()  [unwired: 2 in, 2 out]
            n238 = property on="Задать текущее положение нулевым" class="Bool"("DisabledEnum"=T3."Enabled" ("Disabled")) -> ()  [unwired: 2 in, 2 out]
            n239 = property on="Минуты" class="DigNum (strict)"("DisabledEnum"=T3."Enabled" ("Disabled")) -> ()  [unwired: 2 in, 2 out]
            n240 = property on="положение шд" class="Knob (strict)"("DisabledEnum"=T3."Enabled" ("Disabled")) -> ()  [unwired: 2 in, 2 out]
            n241 = property on="положение в минутах 1" class="Str"("DisabledEnum"=T3."Enabled" ("Disabled")) -> ()  [unwired: 2 in, 2 out]
          }
          frame True {
            n242 = property on="Вернуться в нулевое положение" class="Bool"("DisabledEnum"=T3."Disabled and Grayed Out" ("Disabled")) -> ()  [unwired: 2 in, 2 out]
            n243 = property on="положение шд" class="Knob (strict)"("DisabledEnum"=T3."Disabled and Grayed Out" ("Disabled")) -> ()  [unwired: 2 in, 2 out]
            n244 = property on="текущее положение" class="Str"("DisabledEnum"=T3."Disabled and Grayed Out" ("Disabled")) -> ()  [unwired: 2 in, 2 out]
            n245 = property on="Stop двигатель" class="Bool"("DisabledEnum"=T3."Disabled and Grayed Out" ("Disabled")) -> ()  [unwired: 2 in, 2 out]
            n246 = property on="Вращение по градусам +" class="Bool"("DisabledEnum"=T3."Disabled and Grayed Out" ("Disabled")) -> ()  [unwired: 2 in, 2 out]
            n247 = property on="Вращение по градусам -" class="Bool"("DisabledEnum"=T3."Disabled and Grayed Out" ("Disabled")) -> ()  [unwired: 2 in, 2 out]
            n248 = property on="Задать текущее положение нулевым" class="Bool"("DisabledEnum"=T3."Disabled and Grayed Out" ("Disabled")) -> ()  [unwired: 2 in, 2 out]
            n249 = property on="Минуты" class="DigNum (strict)"("DisabledEnum"=T3."Disabled and Grayed Out" ("Disabled")) -> ()  [unwired: 2 in, 2 out]
            n250 = property on="Установка минут" class="Bool"("DisabledEnum"=T3."Disabled and Grayed Out" ("Disabled")) -> ()  [unwired: 2 in, 2 out]
            n251 = property on="положение в минутах 1" class="Str"("DisabledEnum"=T3."Disabled and Grayed Out" ("Disabled")) -> ()  [unwired: 2 in, 2 out]
          }
        }
      }
      n252 = Close File(refnum=w51) -> ()  [unwired: 1 in, 2 out]
    }
  }
